vi "Lab12_LabView.vi"() -> ()   [LabVIEW 2022 SP3]
uses:
  <vilib>/Instr/_visa.llb/VISA Configure Serial Port (Instr).vi
panel:
  out "LED 8":bool
  out "LED 6":bool
  out "LED 5":bool
  out "LED 3":bool
  out "LED 7":bool
  out "LED 4":bool
  in  "stop":bool
  in  "VISA resource name":refnum<visa-resource-name>
  out "LED 2":bool
  out "LED 1":bool
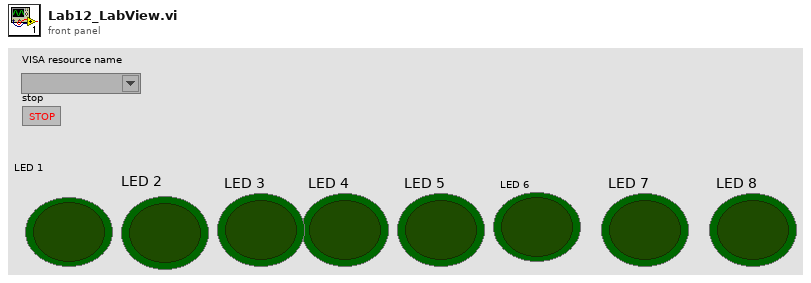
[diagram p1: front panel]
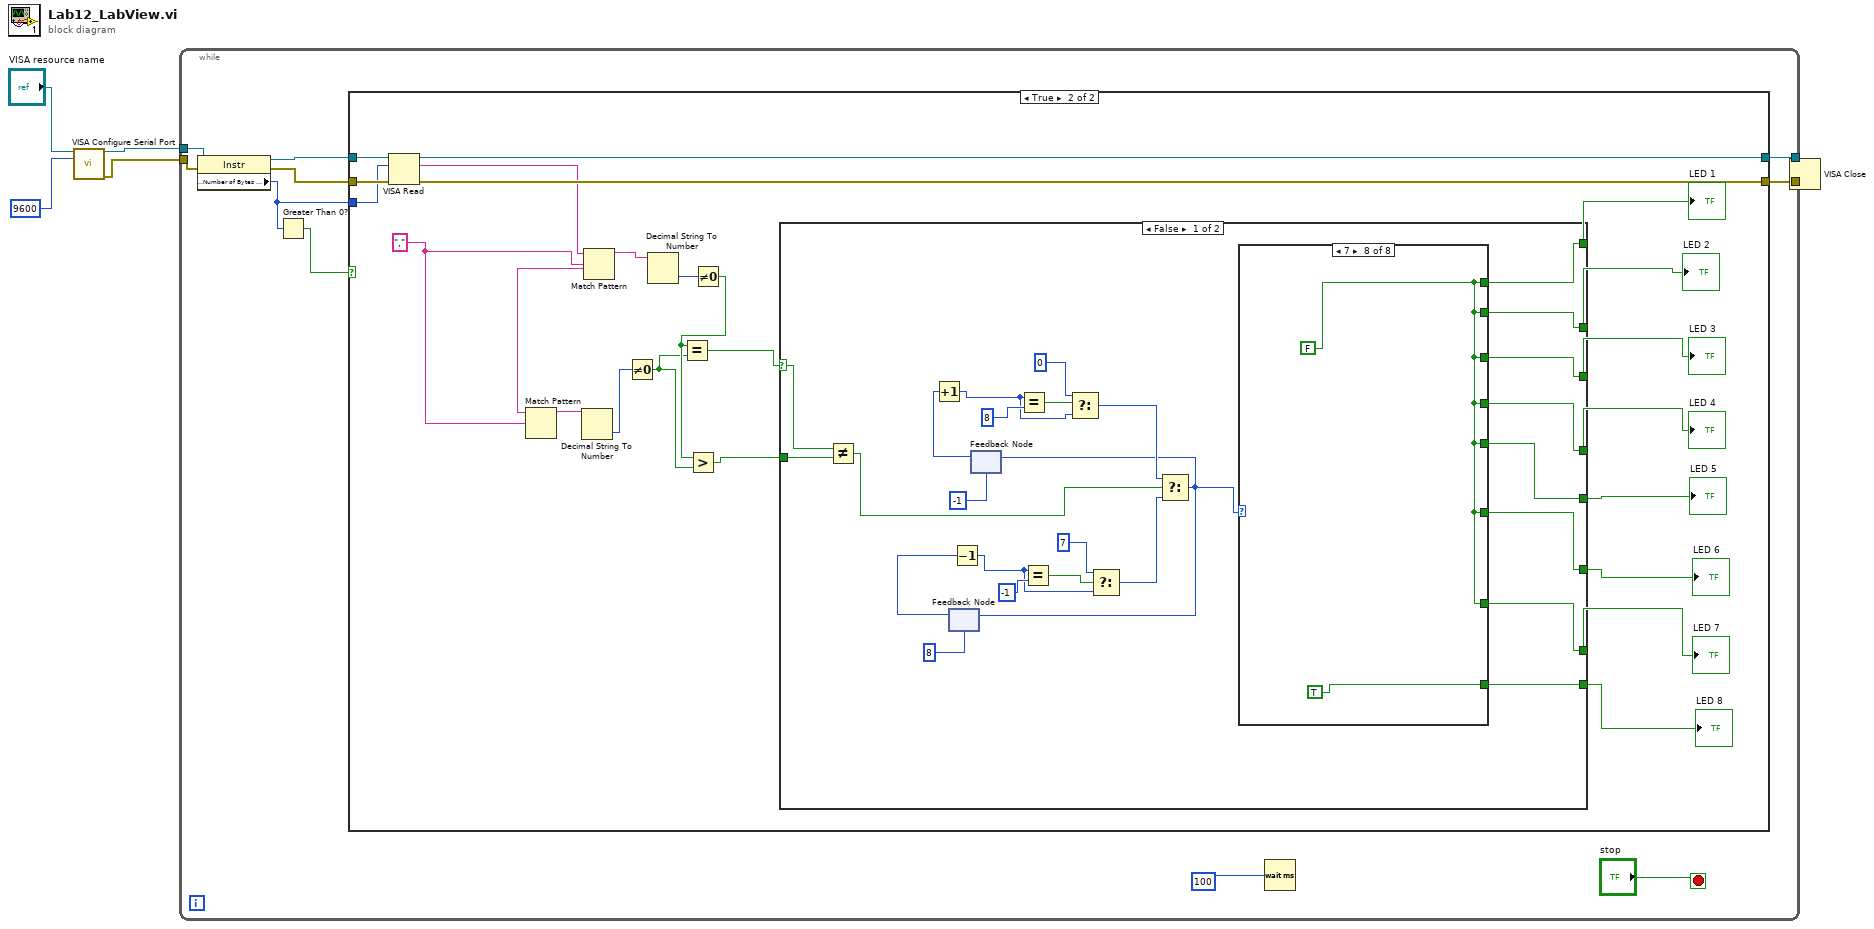
[diagram p0: block diagram]
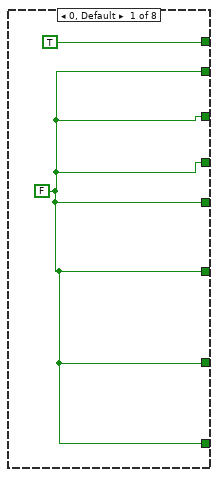
[diagram p3: hidden frame]
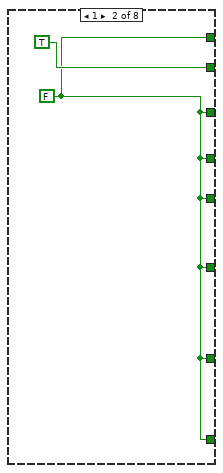
[diagram p4: hidden frame]
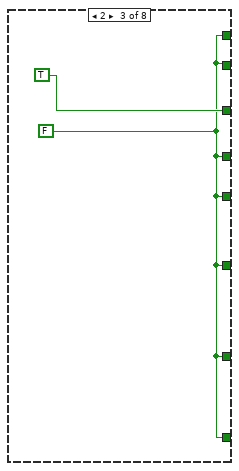
[diagram p5: hidden frame]
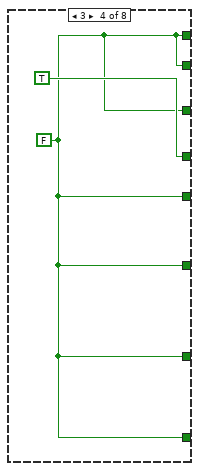
[diagram p6: hidden frame]
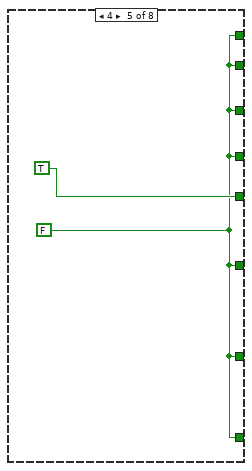
[diagram p7: hidden frame]
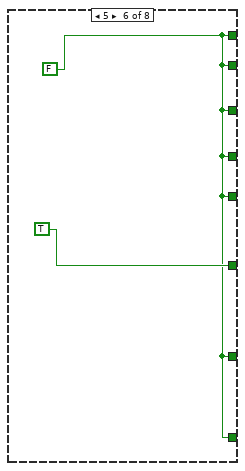
[diagram p8: hidden frame]
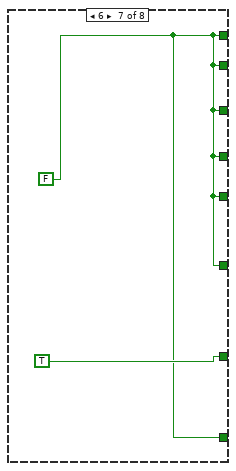
[diagram p9: hidden frame]
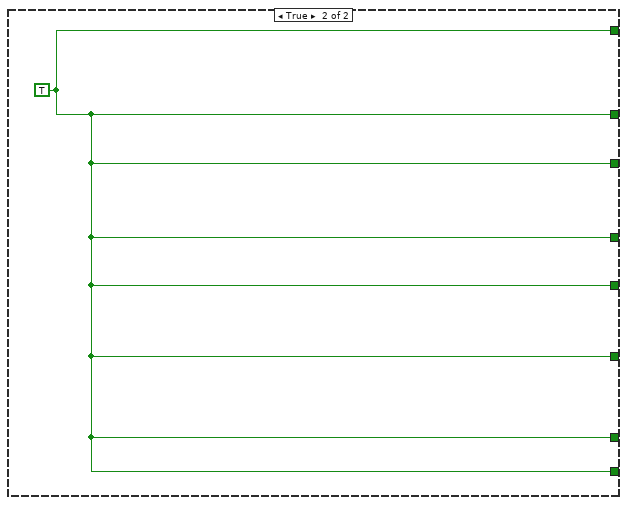
[diagram p10: hidden frame]
diagram:
  n1 = call-poly "VISA Configure Serial Port"("VISA resource name"="VISA resource name", "baud rate (9600)"=u32 9600) -> ("VISA resource name out"=w6:refnum<visa-resource-name>, "error out"=w4:errorcluster)  [unwired: 12 in]
  n2 = while {
    tunnel: w6 -> [w16]
    tunnel: [w14] -> w5
    tunnel: w4 -> [w13]
    tunnel: [w11] -> w3
    stop <- "stop" stop-if-true
    n3 = property class="Instr"(reference=w16, error in=w13) -> (reference out=w15:refnum<visa-resource-name>, error out=w12:errorcluster, "Serial Settings:Number of Bytes at Serial Port"=w8:u32)
    n4 = Greater Than 0?(x=w8) -> (x > 0?=w9:bool)
    n5 = case shown="True" w9 {
      tunnel: w15 -> [w18 w42]
      tunnel: [w18 w41] -> w14
      tunnel: w12 -> [w17 w40]
      tunnel: [w17 w39] -> w11
      tunnel: w8 -> [_ w38]
      frame False {
      }
      frame True {
        w33 = ","
        n6 = VISA Read(VISA resource name=w42, byte count=w38, error in (no error)=w40) -> (VISA resource name out=w41:refnum<visa-resource-name>, read buffer=w37:string, error out=w39:errorcluster)  [unwired: 1 out]
        n7 = Match Pattern(string=w37, regular expression=w33) -> (before substring=w35:string, after substring=w34:string)  [unwired: 1 in, 2 out]
        n8 = Match Pattern(string=w34, regular expression=w33) -> (before substring=w31:string)  [unwired: 1 in, 3 out]
        n9 = Decimal String To Number(string=w31) -> (number=w32:i32)  [unwired: 2 in, 1 out]
        n10 = Not Equal To 0?(x=w32) -> (x != 0?=w20:bool)
        n11 = Decimal String To Number(string=w35) -> (number=w36:i32)  [unwired: 2 in, 1 out]
        n12 = Not Equal To 0?(x=w36) -> (x != 0?=w21:bool)
        n13 = Equal?(x=w21, y=w20) -> (x = y?=w30:bool)
        n14 = Greater?(x=w21, y=w20) -> (0:w19:bool)
        n15 = case shown="False" w30 {
          selector: w30 -> [w68 _]
          tunnel: [w50 w85] -> w29
          tunnel: [w49 w85] -> w28
          tunnel: [w48 w85] -> w27
          tunnel: [w47 w85] -> w26
          tunnel: [w46 w85] -> w25
          tunnel: [w45 w85] -> w24
          tunnel: [w44 w85] -> w23
          tunnel: [w43 w85] -> w22
          tunnel: w19 -> [w67 _]
          frame False {
            n16 = Not Equal?(x=w68, y=w67) -> (x != y?=w59:bool)
            n17 = feedback #1(8) -> (w57:i32)
            n18 = Decrement(x=w57) -> (x-1=w53:i32)
            n19 = feedback #2(-1) -> (w62:i32)
            n20 = Increment(x=w62) -> (x+1=w61:i32)
            n21 = Equal?(x=w61, y=8) -> (x = y?=w65:bool)
            n22 = Equal?(x=w53, y=-1) -> (x = y?=w55:bool)
            n23 = Select(t=0, s=w65, f=w61) -> (s? t:f=w60:i32)
            n24 = Select(t=7, s=w55, f=w53) -> (s? t:f=w52:i32)
            n25 = Select(t=w60, s=w59, f=w52) -> (s? t:f=w51:i32)
            n26 = feedback-in #1(w51) -> ()
            n27 = feedback-in #2(w51) -> ()
            n28 = case shown="7" w51 {
              tunnel: [TRUE w71 w73 w75 w77 w79 w81 w83] -> w50
              tunnel: [w69 TRUE w73 w75 w77 w79 w81 w83] -> w49
              tunnel: [w69 w71 TRUE w75 w77 w79 w81 w83] -> w48
              tunnel: [w69 w71 w73 TRUE w77 w79 w81 w83] -> w47
              tunnel: [w69 w71 w73 w75 TRUE w79 w81 w83] -> w46
              tunnel: [w69 w71 w73 w75 w77 TRUE w81 w83] -> w45
              tunnel: [w69 w71 w73 w75 w77 w79 TRUE w83] -> w44
              tunnel: [w69 w71 w73 w75 w77 w79 w81 TRUE] -> w43
              frame 0, Default {
                w69 = FALSE
              }
              frame 1 {
                w71 = FALSE
              }
              frame 2 {
                w73 = FALSE
              }
              frame 3 {
                w75 = FALSE
              }
              frame 4 {
                w77 = FALSE
              }
              frame 5 {
                w79 = FALSE
              }
              frame 6 {
                w81 = FALSE
              }
              frame 7 {
                w83 = FALSE
              }
            }
          }
          frame True {
            w85 = TRUE
          }
        }
        "LED 1" <- w29
        "LED 2" <- w28
        "LED 4" <- w26
        "LED 7" <- w23
        "LED 5" <- w25
        "LED 6" <- w24
        "LED 8" <- w22
        "LED 3" <- w27
      }
    }
    n29 = Wait (ms)(milliseconds to wait=u32 100) -> ()  [unwired: 1 out]
  }
  n30 = VISA Close(VISA resource name=w5, error in (no error)=w3) -> ()  [unwired: 1 out]
